vi "File Conversion.vi"(1 "Initial File Path":path, 2 "Task":refnum<k21>) -> ()   [LabVIEW 2018]
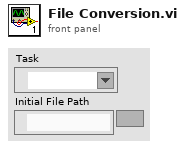
[diagram p1: front panel]
types:
  T1 = enum16{"open", "open or create", "create or replace", "create", "open (read-only)"}
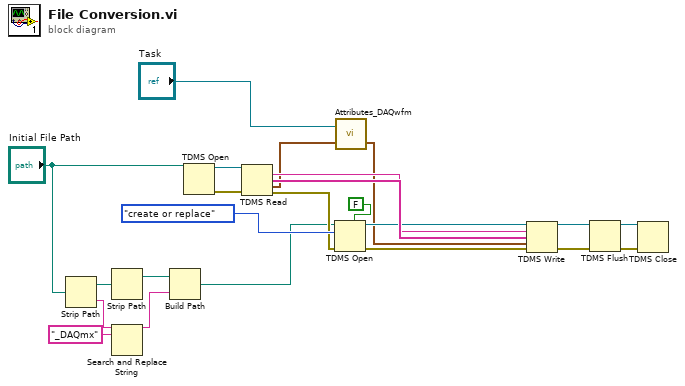
[diagram p0: block diagram]
diagram:
  n1 = Strip Path(path="Initial File Path") -> (stripped path=w6:path, name=w3:string)
  n2 = Strip Path(path=w6) -> (stripped path=w5:path)  [unwired: 1 out]
  n3 = Search and Replace String(input string=w3, search string="_DAQmx") -> (result string=w1:string)  [unwired: 6 in, 3 out]
  n4 = Build Path(base path=w5, name or relative path=w1) -> (appended path=w4:path)
  n5 = TDMS Open(11:"Initial File Path") -> (0:w10:errorcluster, 3:w9:refnum<k34>)  [unwired: 6 in]
  n6 = TDMS Read(0:w9, 11:w10) -> (6:w18:string, 8:w19:string[], 10:w13:waveform(dbl)[], 15:w8:errorcluster)  [unwired: 6 in, 2 out]
  n7 = TDMS Open(5:FALSE ("create index file? (T)"), 8:w8, 10:T1."create or replace" ("operation (0:open)"), 11:w4) -> (0:w17:errorcluster, 3:w16:refnum<k34>)  [unwired: 3 in]
  n8 = call "Attributes_DAQwfm.vi"("data"=w13, "Refnum in"="Task") -> ("Array"=w12:waveform(dbl)[])  [unwired: 1 out]
  n9 = TDMS Write(0:w16, 5:w18, 7:w19, 9:w12, 11:w17) -> (4:w22:refnum<k34>, 15:w23:errorcluster)  [unwired: 1 in, 2 out]
  n10 = TDMS Flush(4:w23, 7:w22) -> (0:w20:errorcluster, 3:w21:refnum<k34>)
  n11 = TDMS Close(8:w20, 11:w21) -> ()  [unwired: 2 out]
